vi "Multiply32.vi"(2 "y":T1 {"mantissa" format="%08x"}, 3 "x":T1 {"mantissa" format="%08x"}) -> (0 "x*y":T1 {"mantissa" format="%08x"})   [LabVIEW 2011]
uses:
  FPGA SGL.ctl
  <vilib>/Platform/TimedLoop/XDataNode/timing_clust.ctl
  <vilib>/Platform/TimedLoop/XDataNode/nitl_modes.ctl
  <vilib>/Platform/TimedLoop/XDataNode/wakeup.ctl
  fpQuantizeFloat.vi
  <vilib>/Platform/TimedLoop/XDataNode/XDataNode.xnode
  <vilib>/rvi/Arithmetic/AddSubMult/XNode/nirviSatArithmetic.xnode
  <vilib>/Platform/TimedLoop/XDataNode/XDNodeRunTimeDep.lvlib
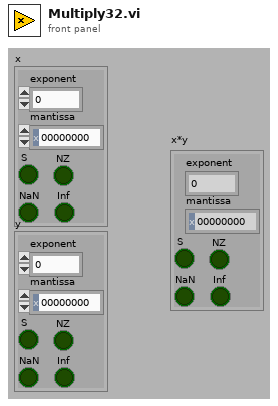
[diagram p1: front panel]
types:
  T1 = typedef "FPGA SGL.ctl" = cluster{"exponent":u8, "mantissa":u32, "S":bool, "NZ":bool, "NaN":bool, "Inf":bool}
  T2 = typedef "XDNodeRunTimeDep.lvlib/timing_clust.ctl" = cluster{"Expected End [f-1]":u64, "Actual End [f-1]":u64, "Finished Late? [f-1]":bool, "Expected End [i-1]":u64, "Actual End [i-1]":u64, "Finished Late? [i-1]":bool, "Expected Start [i]":u64, "Actual Start [i]":u64, "Expected Start [f]":u64, "Actual Start [f]":u64, "Source Name":string, "Structure Name":string, "Period":i64, "Deadline":i64, "Offset":i64, "Start":i64, "Priority":i32, "Timeout":i32, "Mode":T3, "Wakeup Reason":T4, "Error":errorcluster, "Source Type":string, "Secondary Source Type":string, "Global End Time":u64, "Global Start Time":u64, "Frame Duration":u64, "Iteration Duration":u64, "Assigned CPU":i32, "I/O Scan Engine Mode":u32}
  T3 = typedef "XDNodeRunTimeDep.lvlib/nitl_modes.ctl" = enum32{"No Change", "Process missed periods, maintain original phase", "Discard missed periods, maintain original phase", "Process missed periods, ignore original phase", "Discard missed periods, ignore original phase"}
  T4 = typedef "XDNodeRunTimeDep.lvlib/wakeup.ctl" = enum32{"Normal", "Aborted", "Asynchronous wakeup", "Timing source error", "Timed loop error", "Timeout"}
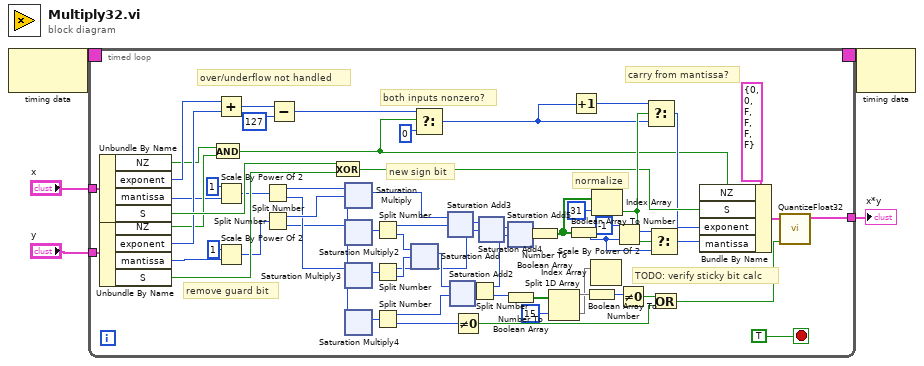
[diagram p0: block diagram]
diagram:
  n1 = node-c288() -> (w1:T2)  [unwired: 1 in]
  n2 = timed-loop {
    tunnel: [w23] -> w3
    tunnel: "y" -> [w60]
    tunnel: "x" -> [w62]
    timing-out: [_] -> w2
    timing: w1 -> [_]
    stop <- TRUE stop-if-true
    # "TODO: verify sticky bit calc"
    # "remove guard bit"
    # "over/underflow not handled"
    # "normalize"
    # "carry from mantissa?"
    # "both inputs nonzero?"
    # "new sign bit"
    n3 = Unbundle By Name(w62) -> ("NZ"=w56:bool, "exponent"=w58:u8, "mantissa"=w49:u32, "S"=w61:bool)
    n4 = Unbundle By Name(w60) -> ("NZ"=w55:bool, "exponent"=w57:u8, "mantissa"=w48:u32, "S"=w59:bool)
    n5 = And(x=w56, y=w55) -> (x .and. y?=w52:bool)
    n6 = Add(x=w58, y=w57) -> (x+y=w22:u8)
    n7 = Scale By Power Of 2(n=1, x=w49) -> (x*2^n=w19:u32)
    n8 = Scale By Power Of 2(n=1, x=w48) -> (x*2^n=w18:u32)
    n9 = Split Number(x=w19) -> (hi(x)=w47:u16, lo(x)=w44:u16)
    n10 = Split Number(x=w18) -> (hi(x)=w46:u16, lo(x)=w43:u16)
    n11 = Subtract(x=w22, y=u8 127) -> (x-y=w20:u8)
    n12 = Exclusive Or(1:w59, 2:w61) -> (0:w54:bool)
    n13 = xnode ("Saturation Multiply")("x"=w47, "y"=w46) -> ("x*y"=w15:u32)
    n14 = xnode ("Saturation Multiply2")("x"=w43, "y"=w47) -> ("x*y"=w41:u32)
    n15 = xnode ("Saturation Multiply3")("x"=w44, "y"=w46) -> ("x*y"=w42:u32)
    n16 = xnode ("Saturation Multiply4")("x"=w44, "y"=w43) -> ("x*y"=w40:u32)
    n17 = Split Number(x=w41) -> (hi(x)=w14:u16, lo(x)=w39:u16)
    n18 = Split Number(x=w42) -> (hi(x)=w12:u16, lo(x)=w38:u16)
    n19 = Split Number(x=w40) -> (hi(x)=w36:u16, lo(x)=w34:u16)
    n20 = xnode ("Saturation Add")("x"=w39, "y"=w38) -> ("x+y"=w37:u32)
    n21 = Select(t=w20, s=w52, f=i8 0) -> (s? t:f=w63:u8)
    n22 = xnode ("Saturation Add3")("x"=w15, "y"=w14) -> ("x+y"=w13:u32)
    n23 = xnode ("Saturation Add2")("x"=w37, "y"=w36) -> ("x+y"=w35:u32)
    n24 = Not Equal To 0?(x=w34) -> (x != 0?=w27:bool)
    n25 = Split Number(x=w35) -> (hi(x)=w10:u16, lo(x)=w33:u16)
    n26 = xnode ("Saturation Add4")("x"=w13, "y"=w12) -> ("x+y"=w11:u32)
    n27 = Number To Boolean Array(number=w33) -> (Boolean array=w32:bool[])
    n28 = xnode ("Saturation Add5")("x"=w11, "y"=w10) -> ("x+y"=w9:u32)
    n29 = Number To Boolean Array(number=w9) -> (Boolean array=w65:bool[])
    n30 = Split 1D Array(array=w32, index=15) -> (first subarray=w30:bool[], second subarray=w25:bool[])
    n31 = Boolean Array To Number(Boolean array=w65) -> (number=w6:u32)
    n32 = Increment(x=w63) -> (x+1=w68:u8)
    n33 = Boolean Array To Number(Boolean array=w30) -> (number=w29:u16)
    n34 = Index Array(array=w25) -> ()  [unwired: 1 in, 1 out]
    n35 = Index Array(array=w65, index=i8 31) -> (element=w66:bool)
    n36 = Scale By Power Of 2(n=-1, x=w6) -> (x*2^n=w7:u32)
    n37 = Not Equal To 0?(x=w29) -> (x != 0?=w28:bool)
    n38 = Select(t=w68, s=w66, f=w63) -> (s? t:f=w53:u8)
    n39 = Select(t=w7, s=w66, f=w6) -> (s? t:f=w45:u32)
    n40 = Or(x=w28, y=w27) -> (x .or. y?=w26:bool)
    n41 = Bundle By Name(cluster=T1 {"exponent"=0, "mantissa"=0, "S"=FALSE, "NZ"=FALSE, "NaN"=FALSE, "Inf"=FALSE} ("x"), "NZ"=w52, "S"=w54, "exponent"=w53, "mantissa"=w45) -> (w24:T1)
    n42 = call-poly "QuantizeFloat32.vi"("sticky bit"=w26, "float in"=w24) -> ("float out"=w23:T1)  [unwired: 8 in]
  }
  "x*y" <- w3
  n43 = node-c288(w2) -> ()  [unwired: 1 out]
